vi "cupFinderv5.vi"(11 "image\n in":T1(plugin-control)) -> (0 "WORK FOR GODS SAKE 2":T1(plugin-control), 1 "X-Out":dbl, 2 "CupPosition":T1(plugin-control), 3 "Refnum out":T1(plugin-control), 4 "Y-Out":dbl, 5 "ImgToCrop":T1(plugin-control), 6 "Found Cup":bool)   [LabVIEW 2017]
uses:
  <vilib>/vision/NI_Vision_Development_Module.lvlib
panel:
  out "ROI Descriptor":T2 {"Contours"."Type" items=["No Selection", "Point", "Line", "Rectangle", "Oval", "Polygon", "Freehand Region", "Annulus", "Unused2", "Unused3", "Broken Line", "Freehand Line", "Rotated Rectangle"]}
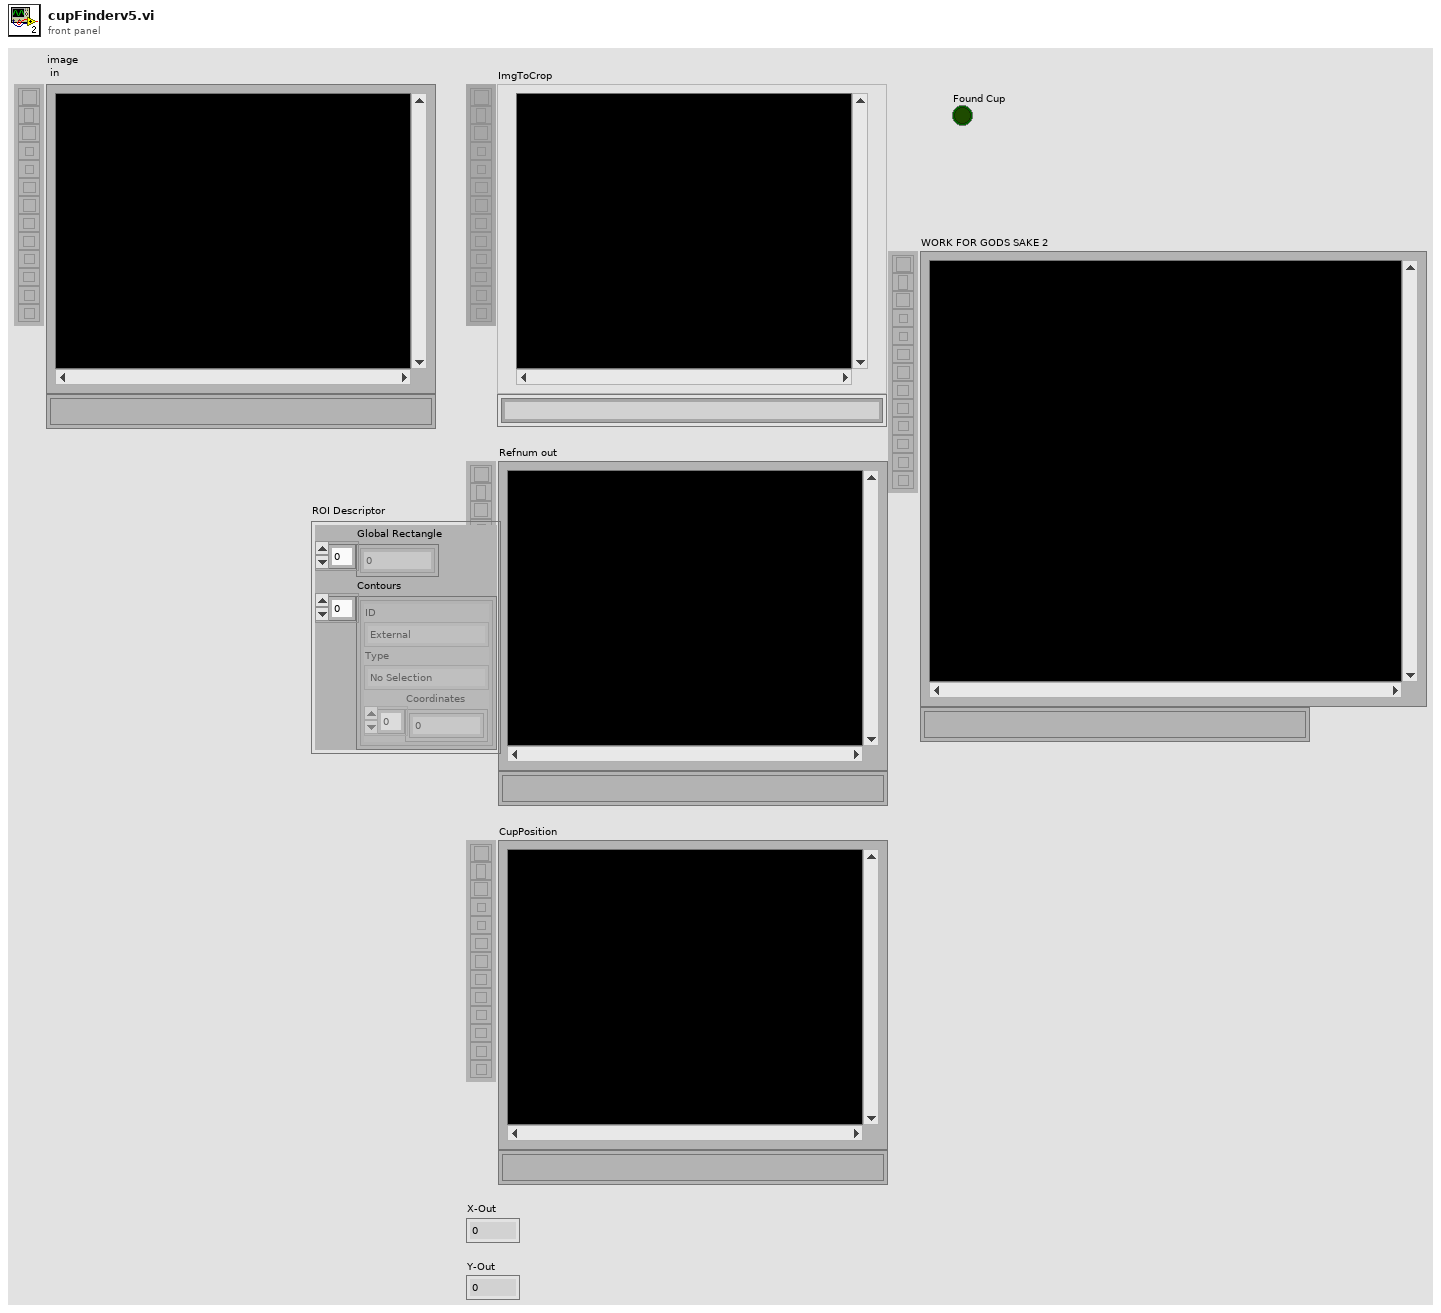
[diagram p1: front panel]
types:
  T1 = typedef "IMAQ Image.ctl" = refnum<image>
  T2 = cluster{"Global Rectangle":i32[], "Contours":cluster{"ID":enum32{"External", "Internal"}, "Type":u32, "Coordinates":i32[]}[]}
  T3 = typedef "Image Type" = u32
  T4 = typedef "IMAQ GM Match Report.ctl" = cluster{"Position":cluster{"x":sgl, "y":sgl}, "Angle":sgl, "Scale":sgl, "Score":sgl, "Bounding Box":cluster{"x":sgl, "y":sgl}[], "Contrast Reversed":bool, "Occlusion %":sgl, "Template Target Curve Score":sgl, "Target Template Curve Score":sgl, "Correlation Score":sgl}
  T5 = typedef "IMAQ Rectangle" = cluster{"Left":i32, "Top":i32, "Right":i32, "Bottom":i32, "Rotation":dbl}
  T6 = typedef "ROI Descriptor" = cluster{"Global Rectangle":i32[], "Contours":cluster{"ID":enum32{"External", "Internal"}, "Type":u32, "Coordinates":i32[]}[]}
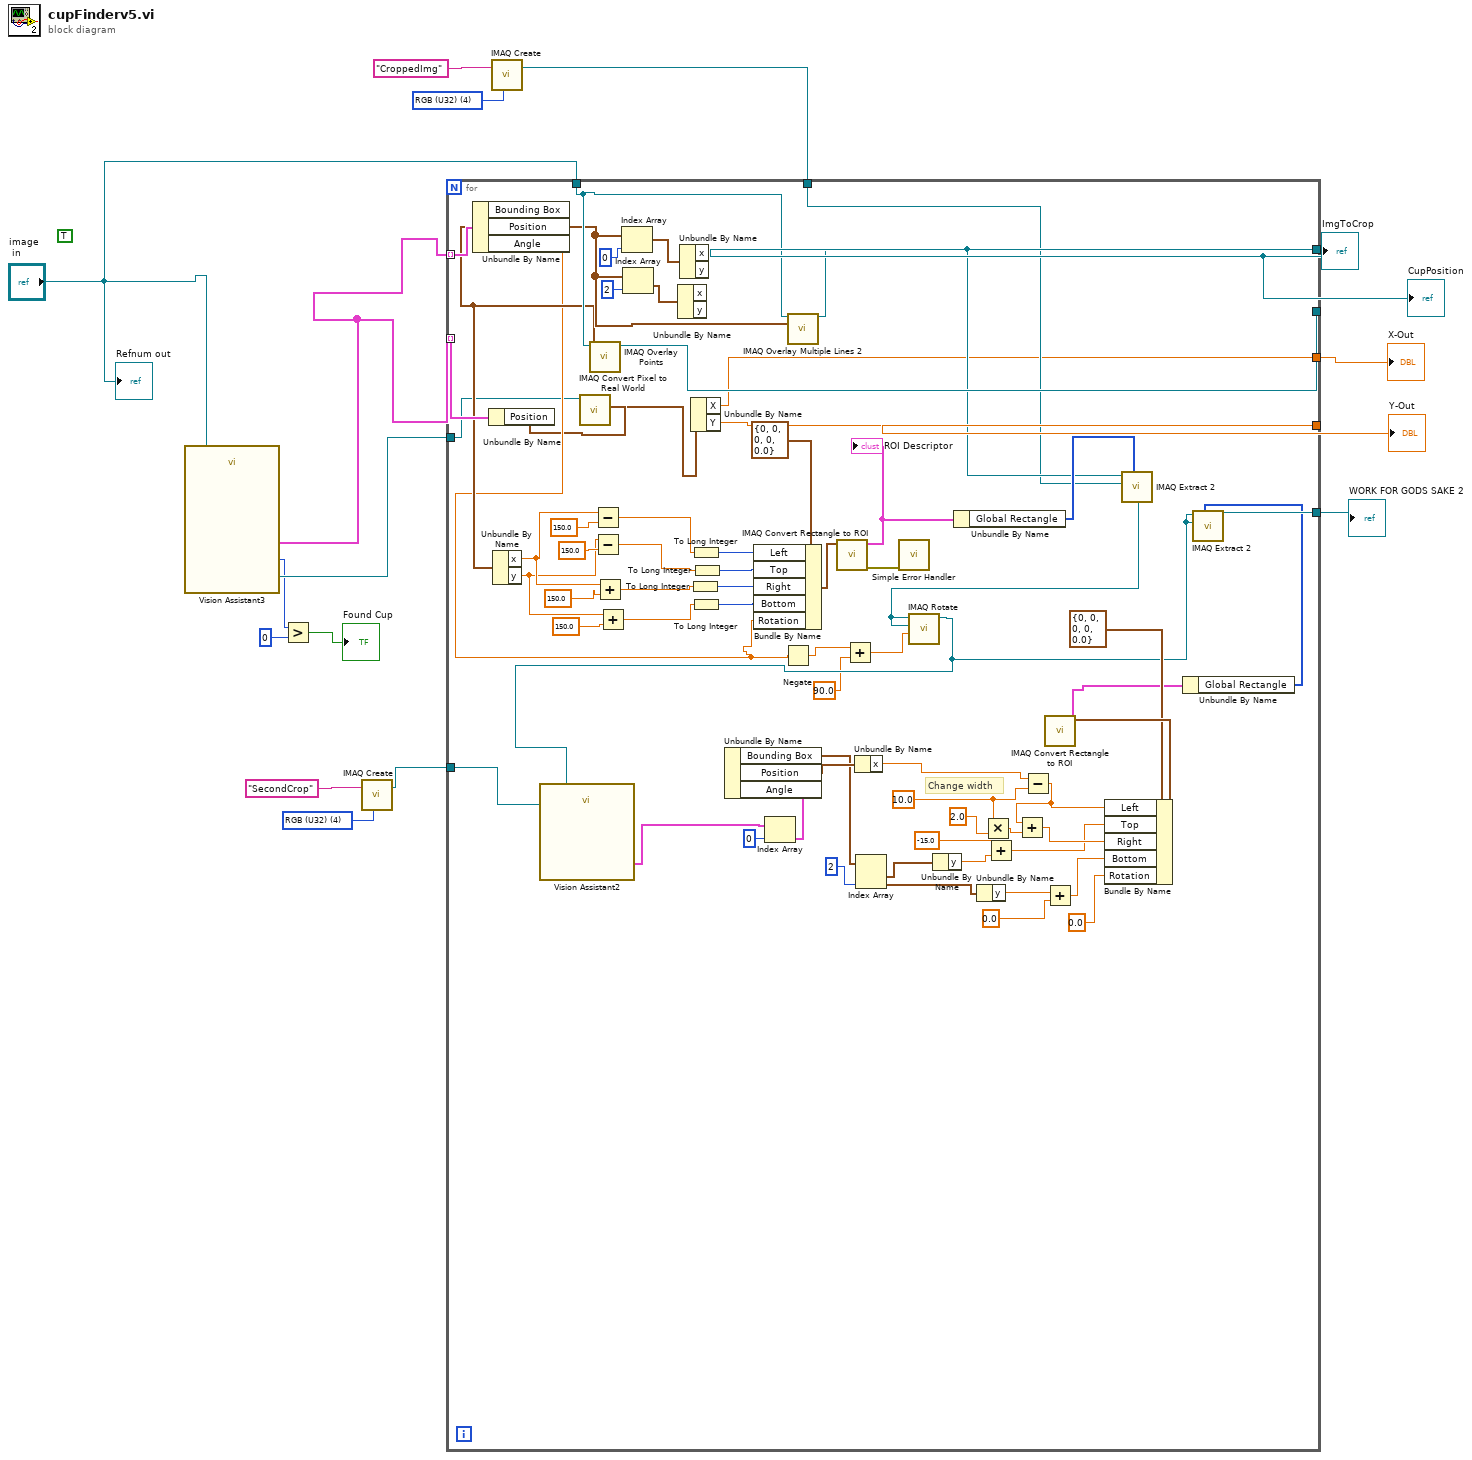
[diagram p0: block diagram]
diagram:
  w9 = T3 4 items=["Grayscale (U8)", "Grayscale (I16)", "Grayscale (SGL)", "Complex (CSG)", "RGB (U32)", "HSL (U32)", "RGB (U64)", "Grayscale (U16)"] ("Image Type")
  w15 = T3 4 items=["Grayscale (U8)", "Grayscale (I16)", "Grayscale (SGL)", "Complex (CSG)", "RGB (U32)", "HSL (U32)", "RGB (U64)", "Grayscale (U16)"] ("Image Type")
  (unwired) TRUE
  n1 = call "Vision Assistant3"("Image In"="image\n in") -> ("Image Out"=w4:T1, "Matches (Geometric Matching 1)"=w5:T4[], "Number of Matches (Geometric Matching 1)"=w3:i32)  [unwired: 23 in, 1 out]
  n2 = Greater?(x=w3, y=0) -> (0:→"Found Cup":bool)
  n3 = call "IMAQ Create"("Image Name"="SecondCrop", "Image Type"=w9) -> ("New Image"=w7:T1)  [unwired: 3 in, 1 out]
  n4 = call "IMAQ Create"("Image Name"="CroppedImg", "Image Type"=w15) -> ("New Image"=w16:T1)  [unwired: 3 in, 1 out]
  n5 = for {
    tunnel: [w67] -> w10
    tunnel: [w85] -> _
    tunnel: [w34] -> w12
    tunnel: [w35] -> w13
    tunnel: "image\n in" -> [w78]
    tunnel: w5 -> [w83] mode=indexing
    tunnel: w5 -> [w84] mode=indexing
    tunnel: w16 -> [w66]
    tunnel: [w54] -> w11
    tunnel: w7 -> [w39]
    tunnel: w4 -> [w38]
    w28 = sgl 10.0 ("y")
    # "Change width"
    n6 = Unbundle By Name(w83) -> ("Bounding Box"=w68:cluster{"x":sgl, "y":sgl}[], "Position"=w65:cluster{"x":sgl, "y":sgl}, "Angle"=w53:sgl)
    n7 = Unbundle By Name(w84) -> ("Position"=w37:cluster{"x":sgl, "y":sgl})
    n8 = Unbundle By Name(w65) -> ("x"=w60:sgl, "y"=w57:sgl)
    n9 = call "IMAQ Convert Pixel to Real World"("Pixel Coordinates"=w37, "Calibrated Image"=w38) -> ("Real World Coordinates"=w36:cluster{"X":sgl, "Y":sgl})  [unwired: 4 in, 5 out]
    n10 = call "IMAQ Overlay Points"("Point"=w65, "Image"=w78) -> ("Image Out"=w85:T1)  [unwired: 8 in, 1 out]
    n11 = Subtract(x=w60, y=sgl 150.0) -> (x-y=w63:sgl)
    n12 = Subtract(x=w57, y=sgl 150.0) -> (x-y=w61:sgl)
    n13 = Add(x=w60, y=sgl 150.0) -> (x+y=w58:sgl)
    n14 = Add(x=w57, y=sgl 150.0) -> (x+y=w55:sgl)
    n15 = Index Array(array=w68, index=0) -> (element=w81:cluster{"x":sgl, "y":sgl})
    n16 = Index Array(array=w68, index=2) -> (element=w79:cluster{"x":sgl, "y":sgl})
    n17 = Unbundle By Name(w79) -> ()  [unwired: 2 out]
    n18 = Unbundle By Name(w81) -> ()  [unwired: 2 out]
    n19 = To Long Integer(number=w58) -> (32bit integer=w73:i32)
    n20 = Unbundle By Name(w36) -> ("X"=w34:sgl, "Y"=w35:sgl)
    n21 = To Long Integer(number=w63) -> (32bit integer=w75:i32)
    n22 = To Long Integer(number=w55) -> (32bit integer=w72:i32)
    n23 = To Long Integer(number=w61) -> (32bit integer=w74:i32)
    n24 = Bundle By Name(cluster=T5 {"Left"=0, "Top"=0, "Right"=0, "Bottom"=0, "Rotation"=0.0} ("Rectangle"), "Left"=w75, "Top"=w74, "Right"=w73, "Bottom"=w72, "Rotation"=w53) -> (w77:T5)
    n25 = Negate(x=w53) -> (-x=w52:sgl)
    n26 = call "IMAQ Overlay Multiple Lines 2"("Image"=w78, "Line End Points"=w68) -> ("Image Out"=w67:T1)  [unwired: 12 in, 1 out]
    n27 = call "IMAQ Convert Rectangle to ROI"("Rectangle"=w77) -> ("error out"=w71:errorcluster, "ROI Descriptor"=w70:T6)  [unwired: 8 in]
    "ROI Descriptor" <- w70
    n28 = Add(x=w52, y=sgl 90.0) -> (x+y=w51:sgl)
    n29 = call <vilib>:"Simple Error Handler.vi"("error in (no error)"=w71) -> ()  [unwired: 4 in, 5 out]
    n30 = Unbundle By Name(w70) -> ("Global Rectangle"=w69:i32[])
    n31 = Multiply(x=w28, y=sgl 2.0) -> (x*y=w29:sgl)
    n32 = call "IMAQ Extract 2"("Optional Rectangle"=w69, "Image Dst"=w66, "Image Src"=w67) -> ("Image Dst Out"=w50:T1)  [unwired: 7 in, 1 out]
    n33 = call "IMAQ Rotate"("Angle (degrees)"=w51, "Image Dst"=w50, "Image Src"=w50) -> ("Image Dst Out"=w42:T1)  [unwired: 7 in, 1 out]
    n34 = call "Vision Assistant2"("Image In"=w42, "Image Dst"=w39) -> ("Matches (Geometric Matching 1)"=w33:T4[])  [unwired: 23 in, 2 out]
    n35 = Index Array(array=w33, index=0) -> (element=w48:T4)
    n36 = Unbundle By Name(w48) -> ("Bounding Box"=w32:cluster{"x":sgl, "y":sgl}[], "Position"=w47:cluster{"x":sgl, "y":sgl})  [unwired: 1 out]
    n37 = Unbundle By Name(w47) -> ("x"=w31:sgl)
    n38 = Index Array(array=w32, index #2=2 ("index")) -> (element #1=w25:cluster{"x":sgl, "y":sgl}, element #2=w24:cluster{"x":sgl, "y":sgl})  [unwired: 1 in]
    n39 = Unbundle By Name(w25) -> ("y"=w21:sgl)
    n40 = Unbundle By Name(w24) -> ("y"=w18:sgl)
    n41 = Add(x=sgl -15.0, y=w21) -> (x+y=w22:sgl)
    n42 = Subtract(x=w31, y=w28) -> (x-y=w30:sgl)
    n43 = Add(x=w30, y=w29) -> (x+y=w26:sgl)
    n44 = Add(x=w18, y=sgl 0.0 ("x")) -> (x+y=w19:sgl)
    n45 = Bundle By Name(cluster=T5 {"Left"=0, "Top"=0, "Right"=0, "Bottom"=0, "Rotation"=0.0} ("Rectangle"), "Left"=w30, "Top"=w22, "Right"=w26, "Bottom"=w19, "Rotation"=0.0) -> (w46:T5)
    n46 = call "IMAQ Convert Rectangle to ROI"("Rectangle"=w46) -> ("ROI Descriptor"=w44:T6)  [unwired: 8 in, 1 out]
    n47 = Unbundle By Name(w44) -> ("Global Rectangle"=w43:i32[])
    n48 = call "IMAQ Extract 2"("Optional Rectangle"=w43, "Image Dst"=w42, "Image Src"=w42) -> ("Image Dst Out"=w54:T1)  [unwired: 7 in, 1 out]
  }
  "ImgToCrop" <- w10
  "CupPosition" <- w10
  "X-Out" <- w12
  "Y-Out" <- w13
  "WORK FOR GODS SAKE 2" <- w11
  "Refnum out" <- "image\n in"
